vi "Contrast Ratio Checker.vi"(6 "Adjust to acceptable?":bool, 9 "On Color":u32(colorbox)=16767232, 10 "Background Color":u32(colorbox)=16767232) -> (1 "Adjusted Color":u32(colorbox)=16767232, 2 "Contrast Ratio":dbl, 3 "Pass?":bool)   [LabVIEW 2021]
doc: "Check to see if the background and oncolor will meet the acceptable ratio for contrast. If not, it will adapt the lightness to try to get into range.\n\nhttps://www.w3.org/WAI/WCAG21/Understanding/contrast-minimum.html\n\n<b>Code Developed By:</b>\nTechnology Service Corporation\n1983 S Liberty Drive\nBloomington, IN 47403\nPhone: 812 558-7100\ncustomtest.tsc.com\n\nDeveloper:\nDaniel Coons"
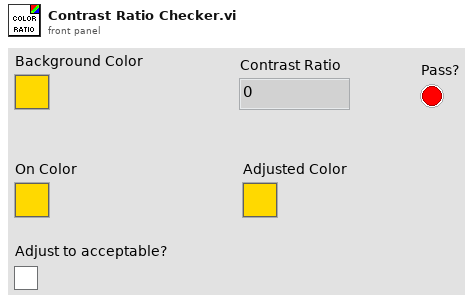
[diagram p1: front panel]
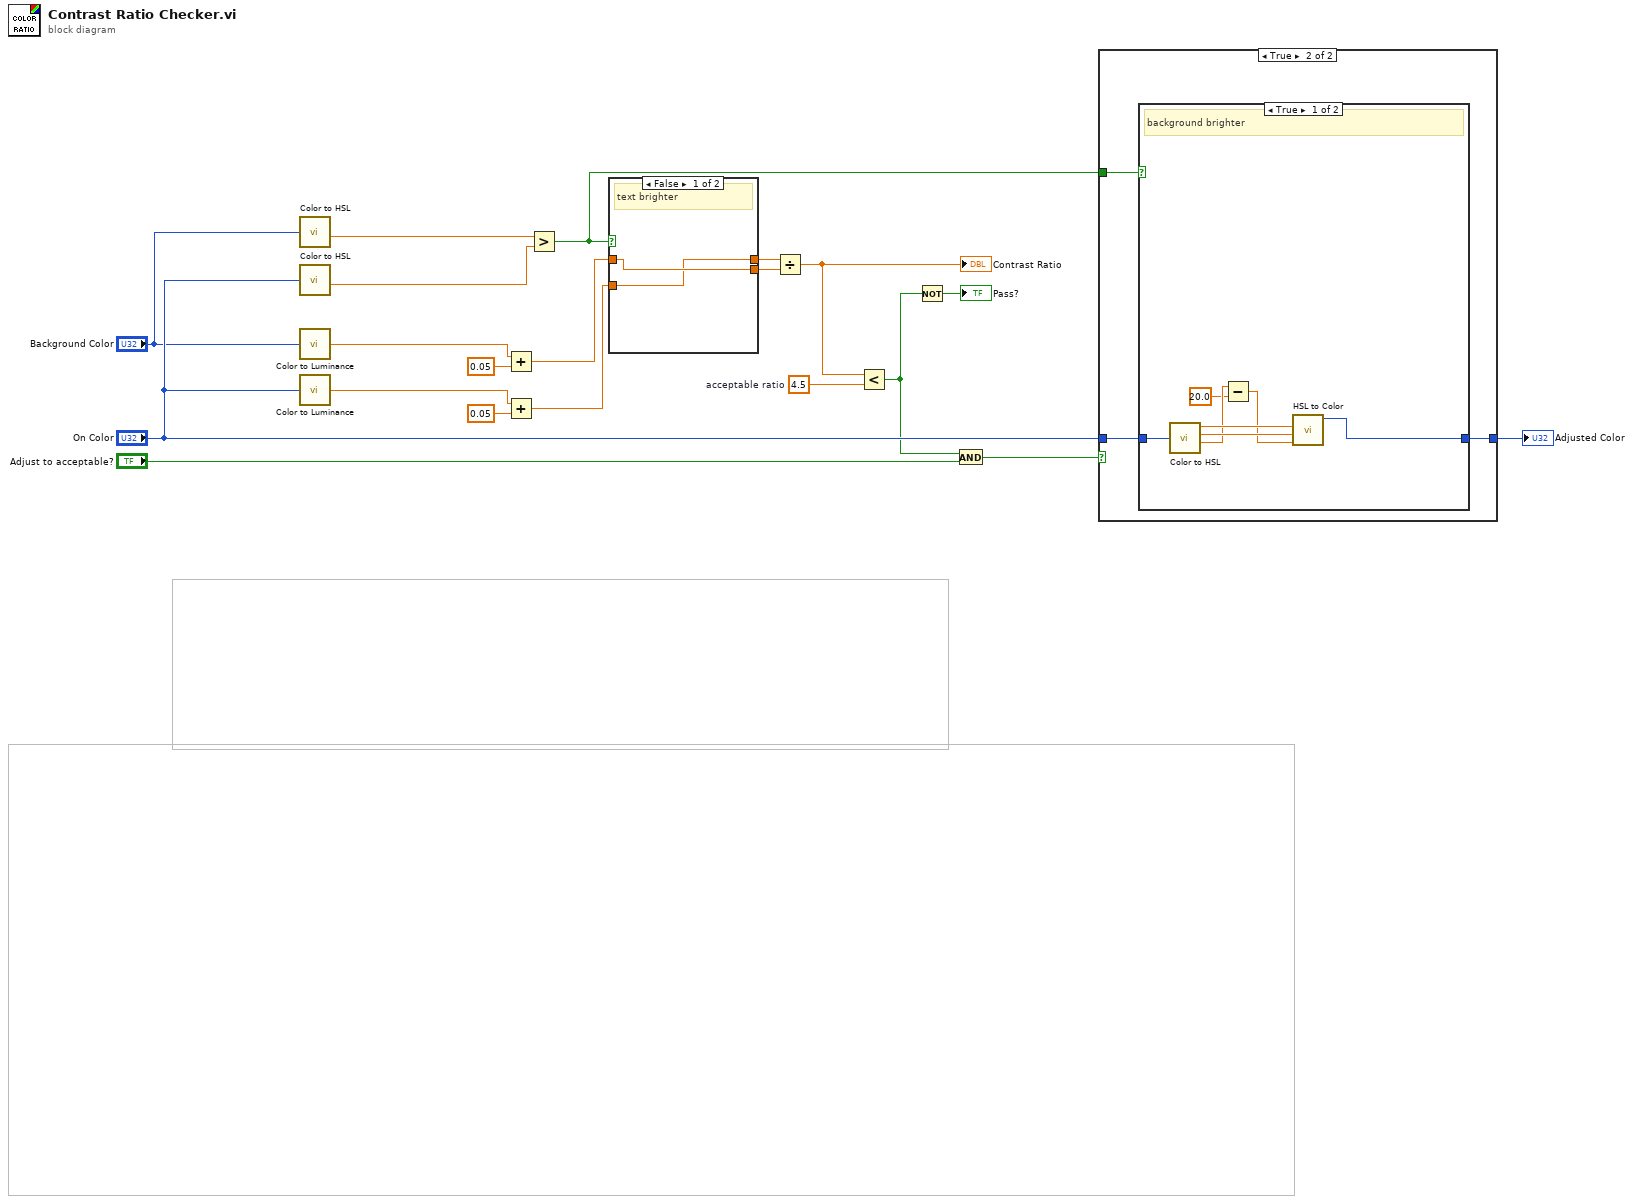
[diagram p0: block diagram]
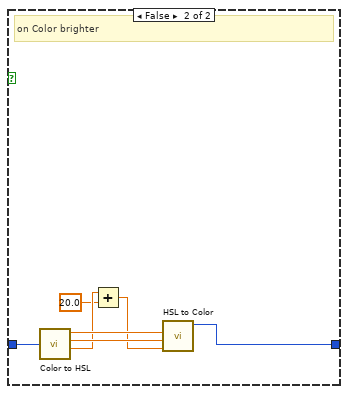
[diagram p3: hidden frame]
diagram:
  w8 = 4.5  # acceptable ratio
  n1 = call "Color to HSL.vi"("Color In"="Background Color") -> ("L (%)"=w20:dbl)  [unwired: 4 in, 3 out]
  n2 = call "Color to HSL.vi"("Color In"="On Color") -> ("L (%)"=w19:dbl)  [unwired: 4 in, 3 out]
  n3 = call "Color to Luminance.vi"("Background Color"="Background Color") -> ("Luminance"=w15:dbl)
  n4 = call "Color to Luminance.vi"("Background Color"="On Color") -> ("Luminance"=w12:dbl)
  n5 = Add(x=w15, y=0.05) -> (x+y=w14:dbl)
  n6 = Add(x=w12, y=0.05) -> (x+y=w11:dbl)
  n7 = Greater?(x=w20, y=w19) -> (0:w3:bool)
  n8 = case shown="False" w3 {
    tunnel: w14 -> [w22 w24]
    tunnel: w11 -> [w21 w23]
    tunnel: [w21 w24] -> w18
    tunnel: [w22 w23] -> w17
    frame False {
      # "text brighter"
    }
    frame True {
      # "background brighter"
    }
  }
  n9 = Divide(x=w18, y=w17) -> (x/y=w9:dbl)
  "Contrast Ratio" <- w9
  n10 = Less?(x=w9, y=w8) -> (x < y?=w5:bool)
  n11 = Not(x=w5) -> (.not. x?=→"Pass?":bool)
  n12 = And(x=w5, y="Adjust to acceptable?") -> (x .and. y?=w7:bool)
  n13 = case shown="True" w7 {
    tunnel: "On Color" -> [w25 w27]
    tunnel: [w25 w26] -> w1
    tunnel: w3 -> [_ w28]
    frame False {
    }
    frame True {
      n14 = case shown="True" w28 {
        tunnel: w27 -> [w35 w42]
        tunnel: [w30 w36] -> w26
        frame True {
          # "background brighter"
          n15 = call "Color to HSL.vi"("Color In"=w35) -> ("H (degrees)"=w34:dbl, "S (%)"=w33:dbl, "L (%)"=w32:dbl)  [unwired: 4 in, 1 out]
          n16 = Subtract(x=w32, y=20.0) -> (x-y=w29:dbl)
          n17 = call "HSL to Color.vi"("L (%)"=w29, "S (%)"=w33, "H (degrees)"=w34) -> ("Color out"=w30:u32)  [unwired: 5 in, 3 out]
        }
        frame False {
          # "on Color brighter"
          n18 = call "Color to HSL.vi"("Color In"=w42) -> ("H (degrees)"=w41:dbl, "S (%)"=w40:dbl, "L (%)"=w39:dbl)  [unwired: 4 in, 1 out]
          n19 = Add(x=w39, y=20.0) -> (x+y=w37:dbl)
          n20 = call "HSL to Color.vi"("L (%)"=w37, "S (%)"=w40, "H (degrees)"=w41) -> ("Color out"=w36:u32)  [unwired: 5 in, 3 out]
        }
      }
    }
  }
  "Adjusted Color" <- w1
